vi "CS_cRIO-PB_DP-Master_ProcessData.vi"(0 "FPGA VI Reference":T2, 7 "Set process data":cluster{"Slave":i32, "Output data":u8[]}[](array[cluster]) {"Output data" format="%.0x"}, 11 "Error":errorcluster) -> (4 "FPGA VI Reference out":T2, 8 "Get process data":T1(array[cluster]) {"Diag data" format="%.0x"; "Output data" format="%.0x"; "Input data" format="%.0x"}, 15 "Error out":errorcluster)   [LabVIEW 2013, in "dynamic profibus.lvlib"]
doc: "Generates a cyclic process image of the connected DP-Slaves.\n\nFPGA VI Reference:\nReference of the FPGA VI.\n\nSet process data:\nThe Set process data array containes the output data for every active DP-Slave. To modify output data, the Output data array for the respective DP-Slave address must to be changed. The output data are shown as array of bytes.\n\nGet process data:\nThe Get process data structure monitors the Input data , the Diag data and the Status for every DP-Slave. The index of the Get process data field complies with the DP-Slave address. The input data are shown as array of bytes. Addionally the DP-Slaves output data are monitored for information purposes.\n\nSlave status:\n0x00: DP-Slave is in DataExchange mode, input and output data are valid\n0xC3: DP-Slave is not in Data Exchange mode, input and output data are invalid, DP-Slave diagnostic data are reported in Diag data array\n0xFF: DP-Slave is in Data Exchange mode and reports ext. diagnostic data, input and output data are valid.\n\nFPGA VI Reference out:\nIs a copy of the FPGA VI Reference .\n\nError in:\nPreceding error conditions. If an error has already occurred, the VI returns the value of the error in Error out.\n\nError out:\nError: TRUE if an error occurred.\nStatus: Error code\nInfo: Error description"
uses:
  dynamic profibus.lvlib
  CS_cRIO-PB_DP-Master_FPGA-Reference.ctl
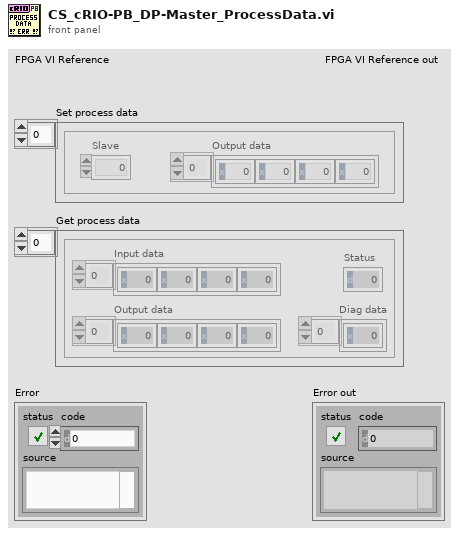
[diagram p1: front panel]
types:
  T1 = cluster{"Status":u8, "Input data":u8[], "Output data":u8[], "Diag data":u8[]}[]
  T2 = typedef "dynamic profibus.lvlib/CS_cRIO-PB_DP-Master_FPGA-Reference.ctl" = refnum<k20>
  T3 = enum16{"Start/Stop DP-Master", "Get Input Data", "Set Output Data", "Get Output Data", "Get Diagnostic Data", "Read/Write Data", "Read Diagnostic Data", "Get DPV1 Data", "Set DPV1 Data", "Read/Write DPV1 Data"}
  T4 = cluster{"Status":u8, "Input data":u8[], "Output data":u8[], "Diag data":u8[]}
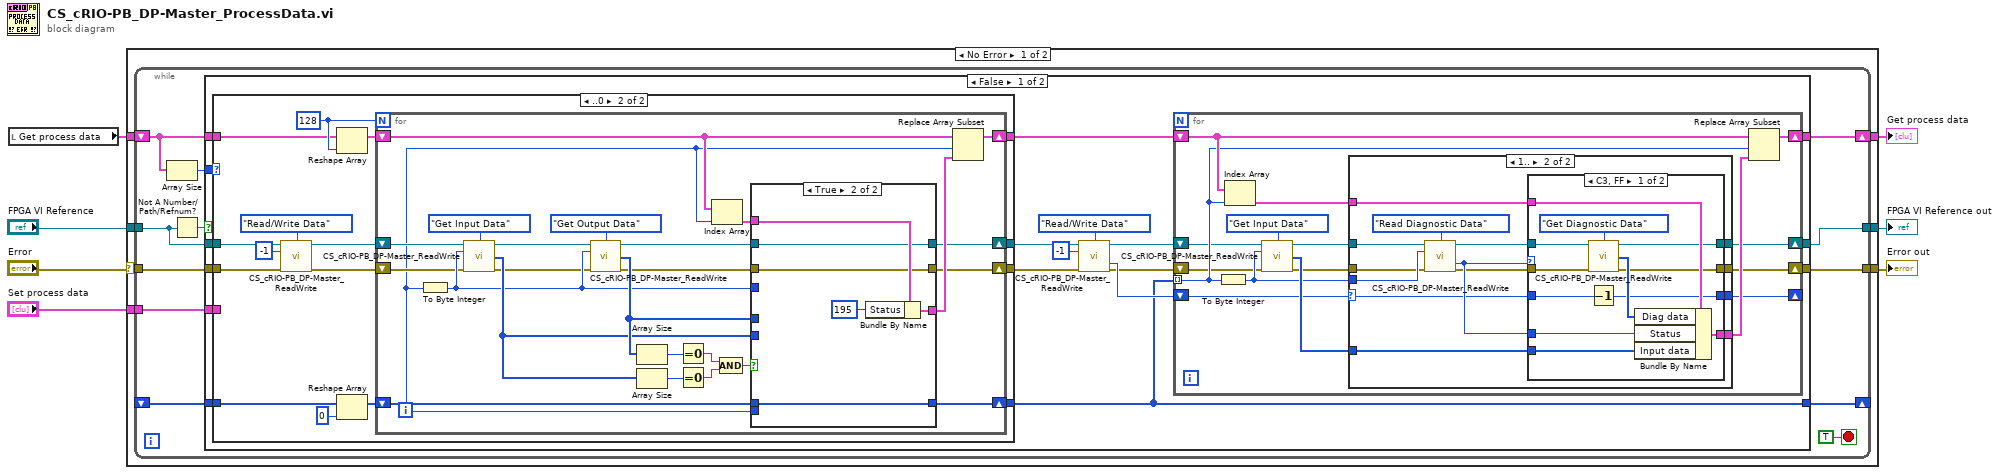
[diagram p0: block diagram]
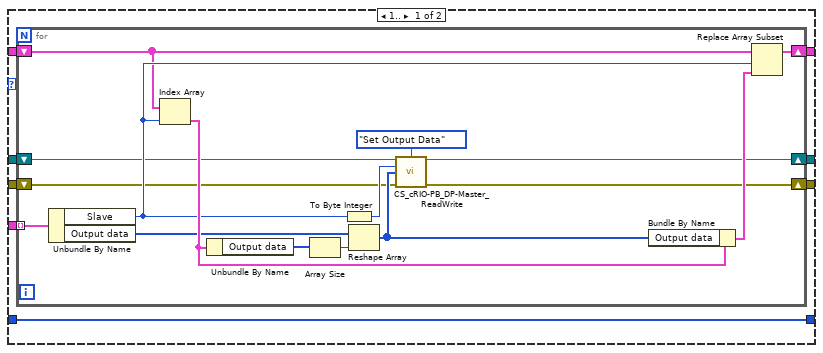
[diagram p2: hidden frame]
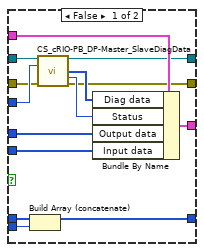
[diagram p3: hidden frame]
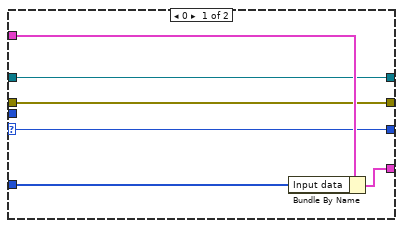
[diagram p4: hidden frame]
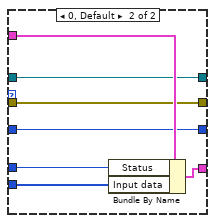
[diagram p5: hidden frame]
diagram:
  n1 = local read "Get process data"() -> (w2:T1)
  n2 = case shown="No Error" "Error" {
    selector: "Error" -> [w13 w187]
    tunnel: "FPGA VI Reference" -> [w14 w188]
    tunnel: [w11 w188] -> w5
    tunnel: [w12 w187] -> w4
    tunnel: "Set process data" -> [w10 _]
    tunnel: w2 -> [w9 _]
    tunnel: [w8 _] -> w1
    frame No Error {
      n3 = while {
        tunnel: w14 -> [w18]
        tunnel: w13 -> [w26]
        tunnel: [w25] -> w12
        tunnel: [w24] -> w11
        tunnel: w10 -> [w23]
        shift-right: [w20] -> w8
        shift-left: w9 -> [w15]
        shift-right: [w21] -> _
        shift-left: _ -> [w22]
        stop <- TRUE stop-if-true
        n4 = Array Size(array=w15) -> (size(s)=w16:i32)
        n5 = Not A Number/Path/Refnum?(number/path/refnum=w18) -> (NaN/Path/Refnum?=w17:bool)
        n6 = case shown="False" w17 {
          tunnel: w26 -> [w43 w186]
          tunnel: [w40 w186] -> w25
          tunnel: [w37 w185] -> w24
          tunnel: w23 -> [w36 _]
          tunnel: w15 -> [w34 _]
          tunnel: w22 -> [w32 _]
          tunnel: [w31 _] -> w21
          tunnel: [w30 _] -> w20
          tunnel: w18 -> [w29 w185]
          tunnel: w16 -> [w28 _]
          frame False {
            n7 = case shown="..0" w28 {
              tunnel: w29 -> [w52 w77]
              tunnel: w43 -> [w51 w78]
              tunnel: [w50 w83] -> w42
              tunnel: [w49 w82] -> w41
              tunnel: w36 -> [w48 _]
              tunnel: [w47 w81] -> w33
              tunnel: w34 -> [w46 w80]
              tunnel: [w45 w73] -> w31
              tunnel: w32 -> [w45 w72]
              frame 1.. {
                n8 = for {
                  tunnel: w48 -> [w62] mode=indexing
                  shift-right: [w63] -> w49
                  shift-left: w52 -> [w65]
                  shift-right: [w64] -> w50
                  shift-left: w51 -> [w54]
                  shift-right: [w60] -> w47
                  shift-left: w46 -> [w61]
                  n9 = Unbundle By Name(w62) -> ("Slave"=w67:i32, "Output data"=w59:u8[])
                  n10 = Index Array(array=w61, index=w67) -> (element=w68:T4)
                  n11 = Unbundle By Name(w68) -> ("Output data"=w57:u8[])
                  n12 = Array Size(array=w57) -> (size(s)=w56:i32)
                  n13 = To Byte Integer(number=w67) -> (8bit integer=w58:i8)
                  n14 = Reshape Array(w59, w56) -> (w55:u8[])
                  n15 = call "CS_cRIO-PB_DP-Master_ReadWrite.vi"("FPGA VI Reference"=w65, "Mode"=T3."Set Output Data", "Slave"=w58, "Data"=w55, "Error"=w54) -> ("FPGA VI Reference out"=w63:T2, "Error out"=w64:errorcluster)  [unwired: 7 in, 2 out]
                  n16 = Bundle By Name(cluster=w68, "Output data"=w55) -> (w66:T4)
                  n17 = Replace Array Subset(array=w61, new element=w66, index=w67) -> (w60:T1)
                }
              }
              frame ..0 {
                w84 = 128
                n18 = call "CS_cRIO-PB_DP-Master_ReadWrite.vi"("FPGA VI Reference"=w77, "Mode"=T3."Read/Write Data", "Slave"=i8 -1 ("-1:ReadWriteProcessData"), "Error"=w78) -> ("FPGA VI Reference out"=w75:T2, "Error out"=w76:errorcluster)  [unwired: 8 in, 2 out]
                n19 = Reshape Array(w80, w84) -> (w74:T1)
                n20 = Reshape Array(w72, 0 ("dimension size")) -> (w71:i32[])
                n21 = for {
                  N: w84 -> [_]
                  shift-right: [w101] -> w82
                  shift-left: w75 -> [w96]
                  shift-right: [w102] -> w83
                  shift-left: w76 -> [w97]
                  shift-right: [w98] -> w81
                  shift-left: w74 -> [w105]
                  shift-right: [w89] -> w73
                  shift-left: w71 -> [w88]
                  i -> [w90]
                  n22 = To Byte Integer(number=w90) -> (8bit integer=w99:i8)
                  n23 = call "CS_cRIO-PB_DP-Master_ReadWrite.vi"("FPGA VI Reference"=w96, "Mode"=T3."Get Input Data", "Slave"=w99, "Error"=w97) -> ("FPGA VI Reference out"=w106:T2, "Data out"=w108:u8[], "Error out"=w95:errorcluster)  [unwired: 8 in, 1 out]
                  n24 = call "CS_cRIO-PB_DP-Master_ReadWrite.vi"("FPGA VI Reference"=w106, "Mode"=T3."Get Output Data", "Slave"=w99, "Error"=w95) -> ("FPGA VI Reference out"=w100:T2, "Data out"=w109:u8[], "Error out"=w94:errorcluster)  [unwired: 8 in, 1 out]
                  n25 = Array Size(array=w109) -> (size(s)=w107:i32)
                  n26 = Array Size(array=w108) -> (size(s)=w87:i32)
                  n27 = Equal To 0?(x=w107) -> (x = 0?=w92:bool)
                  n28 = Equal To 0?(x=w87) -> (x = 0?=w93:bool)
                  n29 = Index Array(array=w105, index=w90) -> (element=w104:T4)
                  n30 = Compound Arithmetic op=AND(w92, w93) -> (w91:bool)
                  n31 = case shown="True" w91 {
                    tunnel: w109 -> [w123 _]
                    tunnel: w104 -> [w122 w129]
                    tunnel: [w119 w128] -> w103
                    tunnel: [w118 w127] -> w102
                    tunnel: [w117 w126] -> w101
                    tunnel: w100 -> [w116 w126]
                    tunnel: w99 -> [w115 _]
                    tunnel: w94 -> [w114 w127]
                    tunnel: w108 -> [w113 _]
                    tunnel: w90 -> [w110 _]
                    tunnel: [w112 w124] -> w89
                    tunnel: w88 -> [w111 w124]
                    frame False {
                      n32 = Build Array (concatenate)(w111, w110) -> (w112:i32[])
                      n33 = call "CS_cRIO-PB_DP-Master_SlaveDiagData.vi"("FPGA VI Reference"=w116, "Slave"=w115, "Error"=w114) -> ("FPGA VI Reference out"=w117:T2, "Diagnostic data"=w121:u8[], "Slave status"=w120:u8, "Error out"=w118:errorcluster)  [unwired: 9 in]
                      n34 = Bundle By Name(cluster=w122, "Diag data"=w121, "Status"=w120, "Output data"=w123, "Input data"=w113) -> (w119:T4)
                    }
                    frame True {
                      n35 = Bundle By Name(cluster=w129, "Status"=u8 195) -> (w128:T4)
                    }
                  }
                  n36 = Replace Array Subset(array=w105, new element=w103, index=w90) -> (w98:T1)
                }
              }
            }
            n37 = call "CS_cRIO-PB_DP-Master_ReadWrite.vi"("FPGA VI Reference"=w41, "Mode"=T3."Read/Write Data", "Slave"=i8 -1 ("-1:ReadWriteProcessData"), "Error"=w42) -> ("FPGA VI Reference out"=w38:T2, "Status"=w44:u8, "Error out"=w39:errorcluster)  [unwired: 8 in, 1 out]
            n38 = for {
              shift-right: [w133] -> w40
              shift-left: w39 -> [w140]
              shift-right: [w134] -> w37
              shift-left: w38 -> [w139]
              shift-right: [w131] -> w30
              shift-left: w33 -> [w144]
              tunnel: w31 -> [w142] mode=indexing
              shift-right: [w135] -> _
              shift-left: w44 -> [w138]
              n39 = To Byte Integer(number=w142) -> (8bit integer=w143:i8)
              n40 = Index Array(array=w144, index=w142) -> (element=w132:T4)
              n41 = call "CS_cRIO-PB_DP-Master_ReadWrite.vi"("FPGA VI Reference"=w139, "Mode"=T3."Get Input Data", "Slave"=w143, "Error"=w140) -> ("FPGA VI Reference out"=w137:T2, "Data out"=w145:u8[], "Error out"=w136:errorcluster)  [unwired: 8 in, 1 out]
              n42 = case shown="1.." w138 {
                selector: w138 -> [w146 w157]
                tunnel: w137 -> [w150 w163]
                tunnel: w136 -> [w149 w162]
                tunnel: [w146 w156] -> w135
                tunnel: [w150 w159] -> w134
                tunnel: [w149 w158] -> w133
                tunnel: w145 -> [w148 w155]
                tunnel: w143 -> [_ w164]
                tunnel: w132 -> [w151 w153]
                tunnel: [w147 w154] -> w141
                frame 0 {
                  n43 = Bundle By Name(cluster=w151, "Input data"=w148) -> (w147:T4)
                }
                frame 1.. {
                  n44 = call "CS_cRIO-PB_DP-Master_ReadWrite.vi"("FPGA VI Reference"=w163, "Mode"=T3."Read Diagnostic Data", "Slave"=w164, "Error"=w162) -> ("FPGA VI Reference out"=w160:T2, "Status"=w165:u8, "Error out"=w161:errorcluster)  [unwired: 8 in, 1 out]
                  n45 = case shown="C3, FF" w165 {
                    tunnel: w161 -> [w174 w180]
                    tunnel: [w173 w180] -> w158
                    tunnel: w160 -> [w175 w178]
                    tunnel: [w172 w178] -> w159
                    tunnel: w157 -> [w171 w179]
                    tunnel: [w170 w179] -> w156
                    tunnel: w165 -> [w169 w183]
                    tunnel: w155 -> [w168 w182]
                    tunnel: [w167 w181] -> w154
                    tunnel: w153 -> [w177 w184]
                    frame 195, 255 {
                      n46 = call "CS_cRIO-PB_DP-Master_ReadWrite.vi"("FPGA VI Reference"=w175, "Mode"=T3."Get Diagnostic Data", "Error"=w174) -> ("FPGA VI Reference out"=w172:T2, "Data out"=w176:u8[], "Error out"=w173:errorcluster)  [unwired: 9 in, 1 out]
                      n47 = Decrement(x=w171) -> (x-1=w170:u8)
                      n48 = Bundle By Name(cluster=w177, "Diag data"=w176, "Status"=w169, "Input data"=w168) -> (w167:T4)
                    }
                    frame 0, Default {
                      n49 = Bundle By Name(cluster=w184, "Status"=w183, "Input data"=w182) -> (w181:T4)
                    }
                  }
                }
              }
              n50 = Replace Array Subset(array=w144, new element=w141, index=w142) -> (w131:T1)
            }
          }
          frame True {
          }
        }
      }
    }
    frame Error {
    }
  }
  "FPGA VI Reference out" <- w5
  "Error out" <- w4
  "Get process data" <- w1
